vi "nanomsg_get_statistic.vi"(3 "error in":errorcluster, 4 "statistic":i32(ring)=101 items=["NN_STAT_ESTABLISHED_CONNECTIONS"=101, "NN_STAT_ACCEPTED_CONNECTIONS"=102, "NN_STAT_DROPPED_CONNECTIONS"=103, "NN_STAT_BROKEN_CONNECTIONS"=104, "NN_STAT_CONNECT_ERRORS"=105, "NN_STAT_BIND_ERRORS"=106, "NN_STAT_ACCEPT_ERRORS"=107, "NN_STAT_CURRENT_CONNECTIONS"=201, "NN_STAT_INPROGRESS_CONNECTIONS"=202, "NN_STAT_CURRENT_EP_ERRORS"=203, "NN_STAT_MESSAGES_SENT"=301, "NN_STAT_MESSAGES_RECEIVED"=302, "NN_STAT_BYTES_SENT"=303, "NN_STAT_BYTES_RECEIVED"=304, "NN_STAT_CURRENT_SND_PRIORITY"=401], 5 "socket in":refnum<class "nanomsg_socket.lvclass">) -> (0 "error out":errorcluster, 1 "result":u64, 2 "socket out":refnum<class "nanomsg_socket.lvclass">)   [LabVIEW 2014, in "nanomsg.lvlib" / "nanomsg_socket.lvclass"]
doc: "Detailed API documentation: http://nanomsg.org/documentation.html"
uses:
  nanomsg_socket.lvclass
  nanomsg_socket.lvclass/nanomsg_socket.ctl
  <vilib>/Utility/error.llb/Error Cluster From Error Code.vi
  nanomsg.lvlib
panel:
  # "NN"
  # "labview"
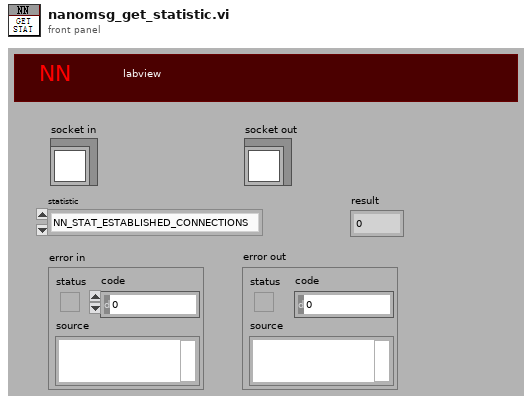
[diagram p1: front panel]
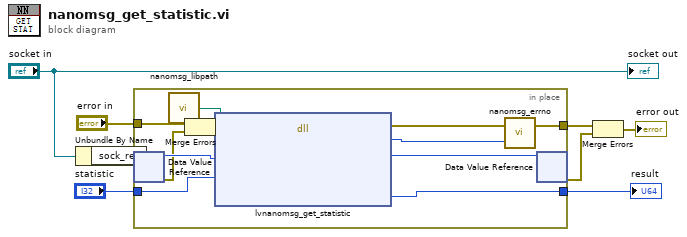
[diagram p0: block diagram]
diagram:
  n1 = Unbundle By Name("socket in") -> ("sock_ref"=w4:refnum<data-value>)
  n2 = in-place {
    in-place-border: "statistic" -> [w19]
    in-place-border: "error in" -> [w18]
    in-place-border: [w16] -> w6
    in-place-border: [w9] -> w1
    n3 = in-place-dvr #1(w4) -> (w15:u64, w11:errorcluster)
    n4 = call "nanomsg_libpath.vi"() -> ("path"=w13:path)
    n5 = Merge Errors(w18, w11) -> (w12:errorcluster)
    n6 = dll-call lib="?" fn="lvnanomsg_get_statistic" ("zmq_labview.dll:lvzmq_connect")(path in=w13, error in=w12, "sock_obj"=w15, "statistic"=w19) -> (error out=w17:errorcluster, "return type"=w10:i32, "sock_obj"=w14:u64, "result"=w9:u64)  [unwired: 3 in, 1 out]
    n7 = call "nanomsg_errno.vi"("retval"=w10, "error in"=w17) -> ("error out"=w16:errorcluster)  [unwired: 1 out]
    n8 = in-place-dvr #1(w14) -> (w2:errorcluster)  [unwired: 1 out]
  }
  "result" <- w1
  n9 = Merge Errors(w6, w2) -> (→"error out":errorcluster)
  "socket out" <- "socket in"
